vi "Initialize HW.vi"(8 "error in (no error)":errorcluster, 11 "DAQmx Servo in":refnum<class "DAQmx Servo.lvclass">) -> (0 "error out":errorcluster, 3 "DAQmx Servo out":refnum<class "DAQmx Servo.lvclass">)   [LabVIEW 2020, in "DAQmx Servo.lvclass"]
uses:
  DAQmx Servo.lvclass
  C:/Users/Haslach/Documents/Inflation-Apparatus/src/Hardware/Actuators/Servos/Servo.lvclass
  C:/Users/Haslach/Documents/Inflation-Apparatus/src/Hardware/General Hardware.lvclass
  Servo.lvclass/Servo.ctl
  General Hardware.lvclass/General Hardware.ctl
  DAQmx Servo.lvclass/DAQmx Servo.ctl
  <vilib>/DAQmx/create/channels.llb/DAQmx Create Channel (CO-Pulse Generation-Frequency).vi
  <vilib>/DAQmx/configure/timing.llb/DAQmx Timing (Implicit).vi
  Servo.lvclass
  General Hardware.lvclass
  C:/Users/Haslach/Documents/Inflation-Apparatus/src/Hardware/Actuators/Actuator.lvclass
  C:/Users/Haslach/Documents/Inflation-Apparatus/src/Hardware/Actuators/Servos/DAQmx Servo/DAQmx Servo.lvclass
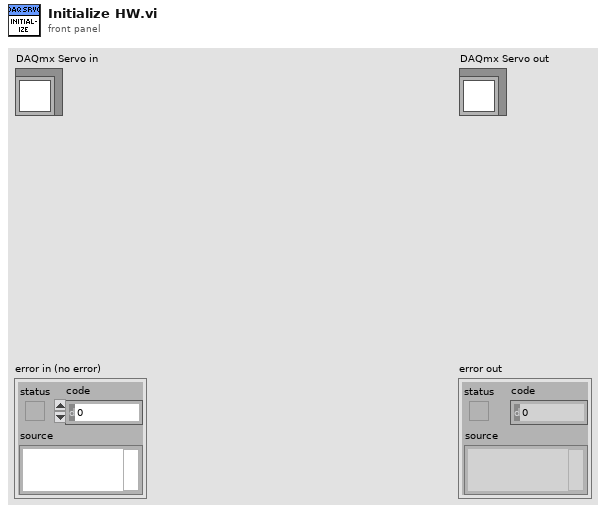
[diagram p1: front panel]
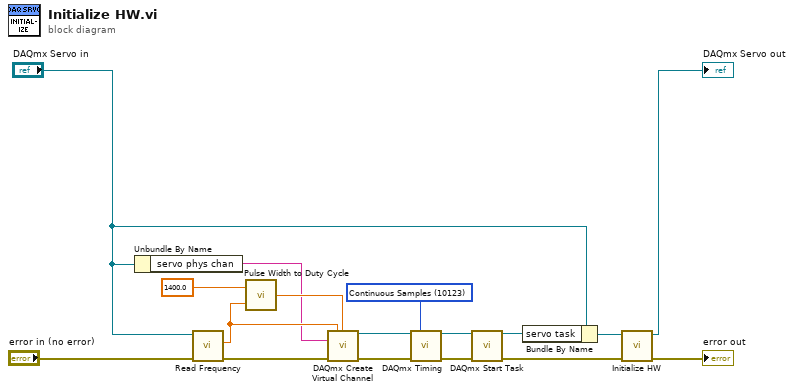
[diagram p0: block diagram]
diagram:
  w12 = 10123 items=["Finite Samples"=10178, "Continuous Samples"=10123, "Hardware Timed Single Point"=12522] ("sample mode")
  n1 = Unbundle By Name("DAQmx Servo in") -> ("servo phys chan"=w7:tag)
  n2 = call "Read Frequency.vi"("error in (no error)"="error in (no error)", "General Hardware in"="DAQmx Servo in") -> ("error out"=w9:errorcluster, "frequency (Hz)"=w8:dbl)  [unwired: 7 in, 1 out]
  n3 = call "Pulse Width to Duty Cycle.vi"("frequency"=w8, "pulse width (us)"=1400.0) -> ("duty cycle"=w10:dbl)
  n4 = call-poly <vilib>:"DAQmx Create Virtual Channel.vi"("frequency"=w8, "duty cycle"=w10, "counter"=w7, "error in"=w9) -> ("task out"=w16:refnum<k21>, "error out"=w15:errorcluster)  [unwired: 10 in]
  n5 = call-poly <vilib>:"DAQmx Timing.vi"("task/channels in"=w16, "sample mode"=w12, "error in"=w15) -> ("task out"=w14:refnum<k21>, "error out"=w13:errorcluster)  [unwired: 11 in]
  n6 = call <vilib>:"DAQmx Start Task.vi"("task/channels in"=w14, "error in"=w13) -> ("task out"=w6:refnum<k21>, "error out"=w11:errorcluster)  [unwired: 12 in]
  n7 = Bundle By Name(cluster="DAQmx Servo in", "servo task"=w6) -> (w5:refnum<class "DAQmx Servo.lvclass">)
  n8 = call-parent "Initialize HW.vi"("error in (no error)"=w11, "Servo in"=w5) -> ("error out"=→"error out":errorcluster, "Servo out"=→"DAQmx Servo out":refnum<class "DAQmx Servo.lvclass">)  [unwired: 8 in]
